vi "ziModGetDoubleData.vi"(8 "Error In":errorcluster, 10 "ModResults":T3, 11 "ModHandle In":T6 {"ModHandle" format="0x%08x"; "Conn" format="0x%08x"}) -> (0 "Error Out":errorcluster, 1 "DoubleSampleGrid":T1[](array[typedef]), 2 "DoubleSample":T2[](array[typedef]), 3 "ModHandle Out":T6 {"ModHandle" format="0x%08x"; "Conn" format="0x%08x"}, 4 "Value":dbl[](array[numeric]))   [LabVIEW 2018, in "Zurich Instruments LabOne.lvlib"]
doc: "Use this vi to get Double Data from a ModResult returned from ziModGetNextNode.vi. It returns an array of Double Data."
uses:
  Zurich Instruments LabOne.lvlib
  Data/ziTypeDoubleDataTS.ctl
  <instrlib>/Zurich Instruments LabOne/Private/ziLV64.framework
  Data/ziTypeDoubleDataTSGrid.ctl
  Data/ziTypePollType.ctl
  ziTypeModHandle.ctl
  ziTypeModResults.ctl
  ziTypeModGenericHeader.ctl
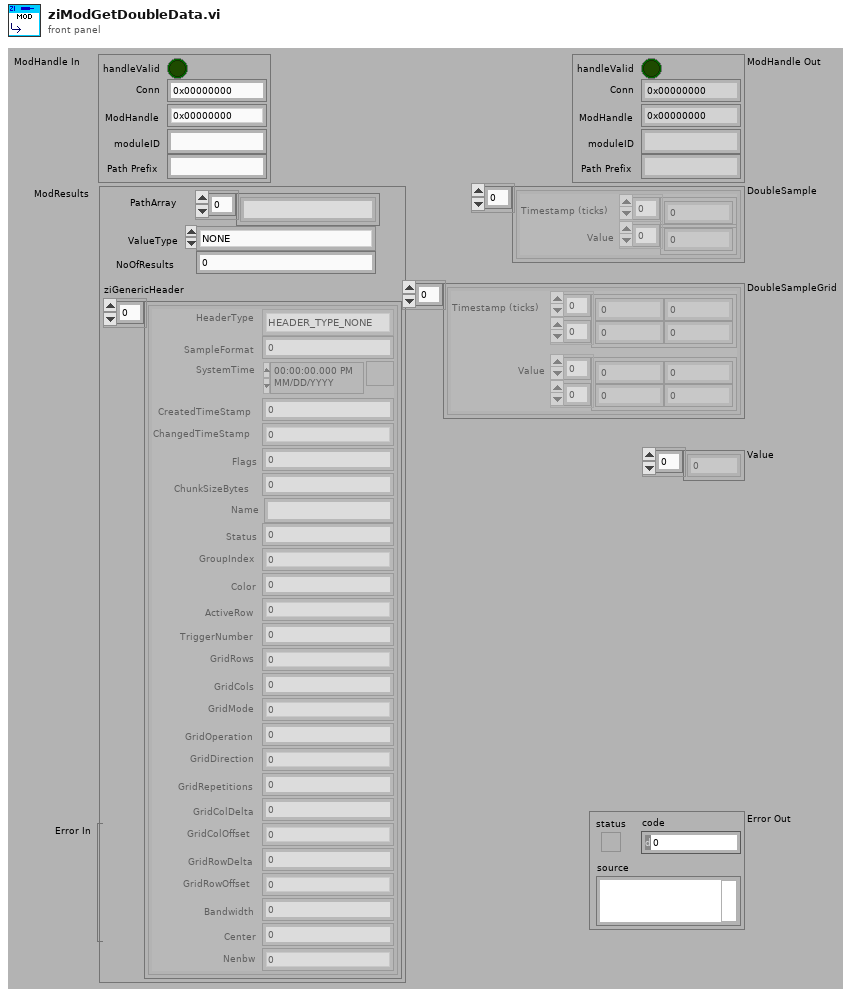
[diagram p1: front panel]
types:
  T1 = typedef "Zurich Instruments LabOne.lvlib/ziTypeDoubleDataTSGrid.ctl" = cluster{"Timestamp (ticks)":u64[][], "Value":dbl[][]}
  T2 = typedef "Zurich Instruments LabOne.lvlib/ziTypeDoubleDataTS.ctl" = cluster{"Timestamp (ticks)":u64[], "Value":dbl[]}
  T3 = typedef "Zurich Instruments LabOne.lvlib/ziTypeModResults.ctl" = cluster{"PathArray":string[], "ValueType":T4, "NoOfResults":u64, "ziGenericHeader":T5[]}
  T4 = typedef "Zurich Instruments LabOne.lvlib/ziTypePollType.ctl" = enum16{"NONE", "DOUBLE_DATA", "INTEGER_DATA", "DEMOD_SAMPLE", "SCOPE_WAVE_HF2", "AUXIN_SAMPLE", "DIO_SAMPLE", "BYTE_ARRAY", "PWA_WAVE", "9", "10", "11", "12", "13", "14", "15", "TREE_CHANGE_DEPRI", "17", "ERROR", "19", "20", "21", "22", "23", "24", "25", "26", "27", "28", "29", "30", "31", "DOUBLE_DATA_TS", "INTEGER_DATA_TS", "34", "SCOPE_WAVE", "SCOPE_WAVE_EX", "37", "BYTE_ARRAY_TS", "39", "40", "41", "42", "43", "44", "45", "CNT_DATA", "47", "TREE_CHANGE", "49", "50", "51", "52", "53", "54", "55", "56", "57", "58", "59", "60", "61", "62", "63", "SWEEPER_DATA", "SPECTRUM_DATA", "ADVISOR_DATA", "VECTOR_DATA", "IMP_DATA"}
  T5 = typedef "Zurich Instruments LabOne.lvlib/ziTypeModGenericHeader.ctl" = cluster{"HeaderType":enum8{"HEADER_TYPE_NONE", "HEADER_TYPE_SWTRIGGER", "HEADER_TYPE_SWEEPER"}, "SampleFormat":u8, "SystemTime":timestamp, "CreatedTimeStamp":u64, "ChangedTimeStamp":u64, "Flags":u32, "ChunkSizeBytes":u64, "Name":string, "Status":u32, "GroupIndex":u32, "Color":u32, "ActiveRow":u32, "TriggerNumber":u64, "GridRows":u32, "GridCols":u32, "GridMode":u32, "GridOperation":u32, "GridDirection":u32, "GridRepetitions":u32, "GridColDelta":dbl, "GridColOffset":dbl, "GridRowDelta":dbl, "GridRowOffset":dbl, "Bandwidth":dbl, "Center":dbl, "Nenbw":dbl}
  T6 = typedef "Zurich Instruments LabOne.lvlib/ziTypeModHandle.ctl" = cluster{"handleValid":bool, "Conn":u64, "ModHandle":u64, "moduleID":string, "Path Prefix":string}
  T7 = cluster{"Timestamp (ticks)":u64[], "Value":dbl[]}
  T8 = cluster{"Timestamp (ticks)":u64[], "Value":i64[]}
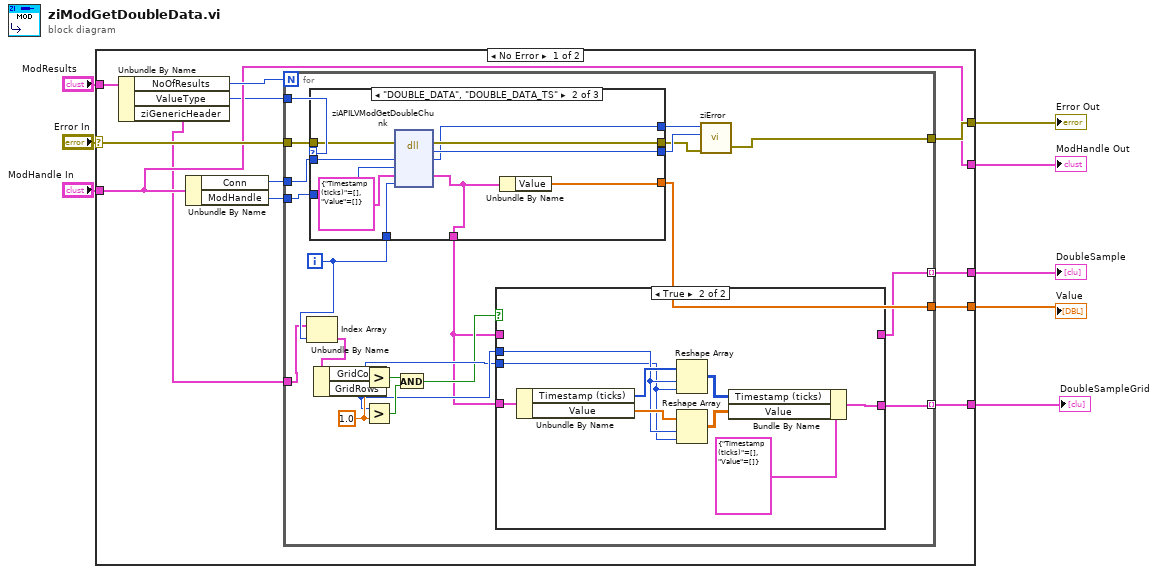
[diagram p0: block diagram]
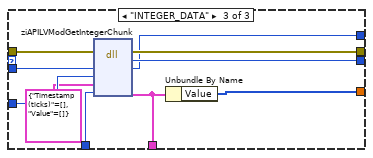
[diagram p4: hidden frame]
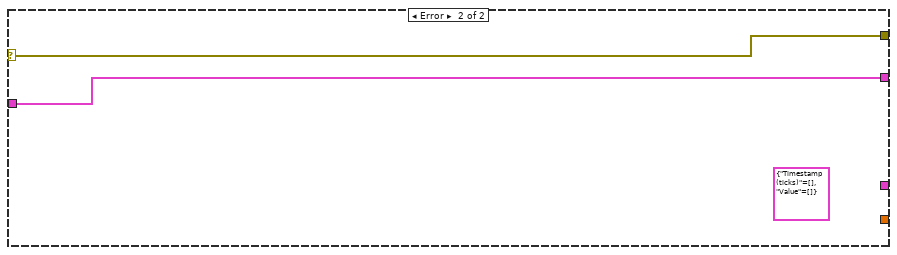
[diagram p5: hidden frame]
diagram:
  n1 = case shown="No Error" "Error In" {
    selector: "Error In" -> [w15 w74]
    tunnel: [w16 w74] -> w4
    tunnel: [w13 w75] -> w7
    tunnel: "ModHandle In" -> [w13 w75]
    tunnel: "ModResults" -> [w18 _]
    tunnel: [w11 _] -> w2
    tunnel: [w14 _] -> w3
    tunnel: [w9 _] -> w1
    frame No Error {
      n2 = Unbundle By Name(w18) -> ("NoOfResults"=w17:u64, "ValueType"=w12:T4, "ziGenericHeader"=w10:T5[])
      n3 = Unbundle By Name(w13) -> ("Conn"=w20:u64, "ModHandle"=w19:u64)
      n4 = for {
        N: w17 -> [_]
        tunnel: w20 -> [w41]
        tunnel: w19 -> [w40]
        tunnel: [w39] -> w16
        tunnel: w15 -> [w36]
        tunnel: [w35] -> w14
        tunnel: w12 -> [w34]
        tunnel: [w25] -> w11 mode=indexing
        tunnel: w10 -> [w22]
        tunnel: [w24] -> w9 mode=indexing
        i -> [w23]
        w32 = 1.0 ("y")
        n5 = Index Array(array=w22, index=w23) -> (element=w21:T5)
        n6 = case shown="\"DOUBLE_DATA\", \"DOUBLE_DATA_TS\"" w34 {
          tunnel: w41 -> [w52 w63 w73]
          tunnel: w40 -> [_ w62 w72]
          tunnel: w23 -> [_ w61 w71]
          tunnel: [_ w60 w70] -> w38
          tunnel: [w53 w59 w69] -> w37
          tunnel: w36 -> [w53 w58 w68]
          tunnel: [_ w56 w67] -> w35
          tunnel: [_ w55 w65] -> w26
          tunnel: [w52 w54 w64] -> w33
          frame "NONE", Default {
          }
          frame "DOUBLE_DATA", "DOUBLE_DATA_TS" {
            n7 = dll-call lib="Applications/National Instruments/LabVIEW 2019 64-bit/instr.lib/Zurich Instruments LabOne/Private/ziLV*.*" fn="ziAPILVModGetDoubleChunk"(error in=w58, "Conn"=w63, "ModHandle"=w62, "DoubleData"=T7 {"Timestamp (ticks)"=[], "Value"=[]} ("DoubleSample"), "chunk_idx"=w61) -> (error out=w59:errorcluster, "return type"=w60:u32, "Conn"=w54:u64, "DoubleData"=w55:T7)  [unwired: 4 in, 1 out]
            n8 = Unbundle By Name(w55) -> ("Value"=w56:dbl[])
          }
          frame "INTEGER_DATA" {
            n9 = dll-call lib="Applications/National Instruments/LabVIEW 2019 64-bit/instr.lib/Zurich Instruments LabOne/Private/ziLV*.*" fn="ziAPILVModGetIntegerChunk"(error in=w68, "Conn"=w73, "ModHandle"=w72, "DoubleData"=T8 {"Timestamp (ticks)"=[], "Value"=[]} ("DoubleSample"), "chunk_idx"=w71) -> (error out=w69:errorcluster, "return type"=w70:u32, "Conn"=w64:u64, "DoubleData"=w65:T8)  [unwired: 4 in, 1 out]
            n10 = Unbundle By Name(w65) -> ("Value"=w67:i64[])
          }
        }
        n11 = Unbundle By Name(w21) -> ("GridCols"=w28:u32, "GridRows"=w29:u32)
        n12 = Greater?(x=w28, y=w32) -> (0:w30:bool)
        n13 = Greater?(x=w29, y=w32) -> (0:w31:bool)
        n14 = And(x=w30, y=w31) -> (x .and. y?=w27:bool)
        n15 = case shown="True" w27 {
          tunnel: w26 -> [_ w51]
          tunnel: w26 -> [w42 _]
          tunnel: [w42 _] -> w25
          tunnel: w29 -> [_ w48]
          tunnel: w28 -> [_ w45]
          tunnel: [_ w47] -> w24
          frame False {
          }
          frame True {
            n16 = Unbundle By Name(w51) -> ("Timestamp (ticks)"=w50:u64[], "Value"=w49:dbl[])
            n17 = Reshape Array(w50, w48, w45) -> (w44:u64[][])
            n18 = Reshape Array(w49, w48, w45) -> (w43:dbl[][])
            n19 = Bundle By Name(cluster=T1 {"Timestamp (ticks)"=[], "Value"=[]} ("DoubleSample"), "Timestamp (ticks)"=w44, "Value"=w43) -> (w47:T1)
          }
        }
        n20 = call "ziError.vi"("Conn"=w33, "ziErrorCode"=w38, "Error In"=w37) -> ("Error Out"=w39:errorcluster)  [unwired: 2 in, 1 out]
      }
    }
    frame Error {
      (unwired) T2 {"Timestamp (ticks)"=[], "Value"=[]} ("DoubleSample")
    }
  }
  "Error Out" <- w4
  "ModHandle Out" <- w7
  "Value" <- w3
  "DoubleSample" <- w2
  "DoubleSampleGrid" <- w1
